vi "Model OPCUA Check Status.vi"(8 "error in (no error)":errorcluster, 11 "Model_AMC in":refnum<class "Model_AMC.lvclass">) -> (0 "error out":errorcluster, 3 "Model_AMC out":refnum<class "Model_AMC.lvclass">)   [LabVIEW 2021, in "Model_AMC.lvclass"]
uses:
  Model_AMC.lvclass
  Model_AMC.lvclass/Model_AMC.ctl
  <userlib>/John_Lib/AMC_FW/AMC_FW.lvlib
  <userlib>/John_Lib/OPCUA/OPCUA.lvclass
  1a8ff785-ae6d-495a-9cae-a72b057f70a7.vi
  d4dfea47-cd05-4011-96e4-e19734fac517.vi
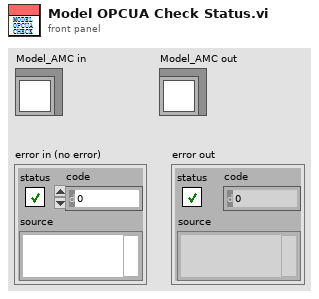
[diagram p1: front panel]
types:
  T1 = typedef "AMC_FW.lvlib/Queue.ctl" = cluster{"Q":T2, "Name":string}
  T2 = typedef "AMC_FW.lvlib/Message Queue.ctl" = refnum<queue>
  T3 = typedef "Model_AMC.lvclass/DVR.ctl" = cluster{"JKI_Network_Streams":refnum<class "NetworkConnection.lvclass">, "AMC Q":T4}
  T4 = typedef "Model_AMC.lvclass/AMC Q.ctl" = cluster{"Main":T1, "OPCUA":T1, "NetworkSteam":T1}
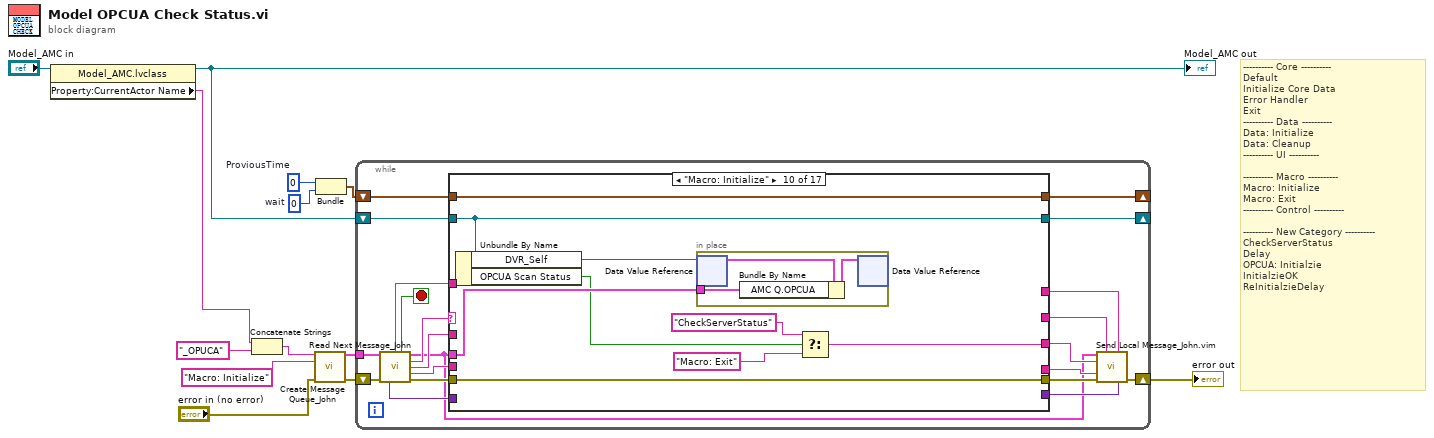
[diagram p0: block diagram]
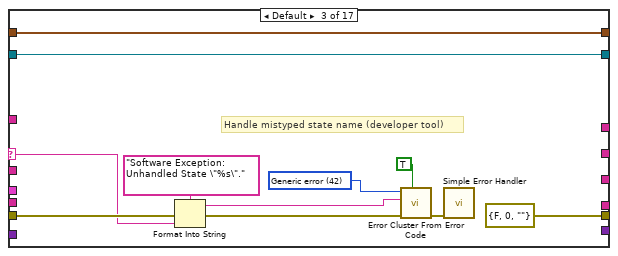
[diagram p4: hidden frame]
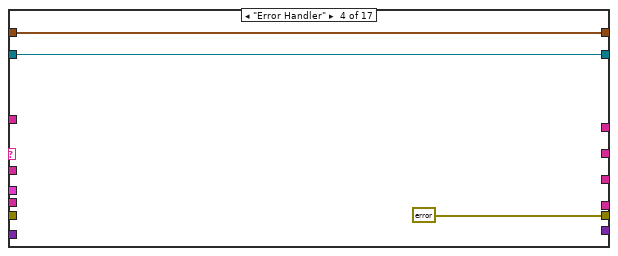
[diagram p5: hidden frame]
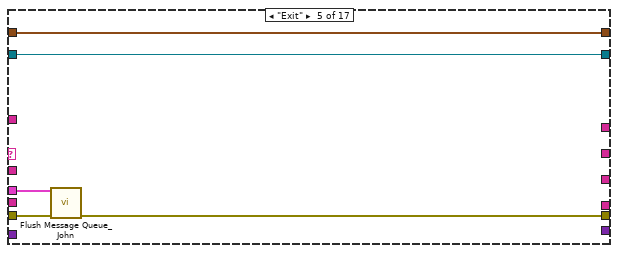
[diagram p6: hidden frame]
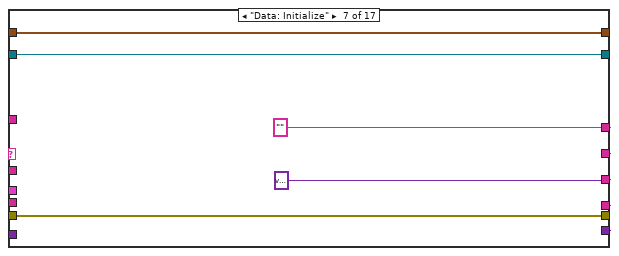
[diagram p8: hidden frame]
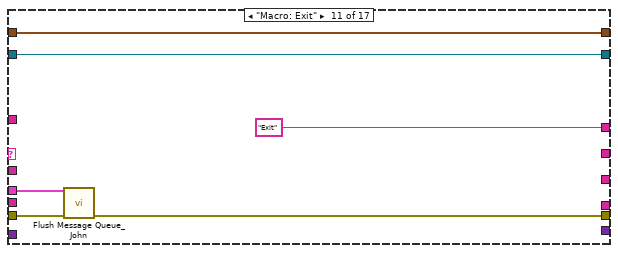
[diagram p11: hidden frame]
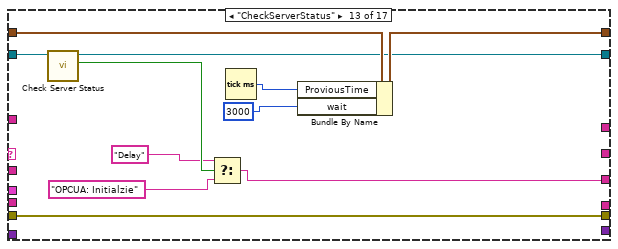
[diagram p13: hidden frame]
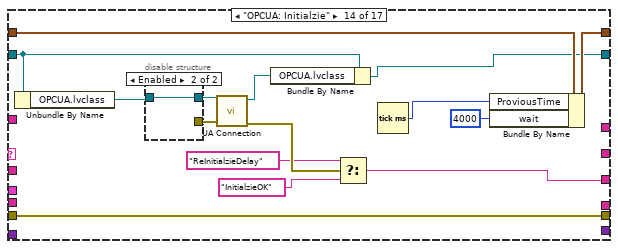
[diagram p14: hidden frame]
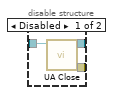
[diagram p15: hidden frame]
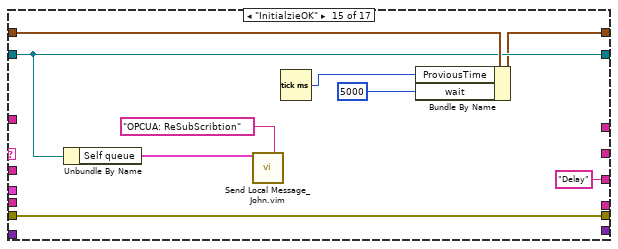
[diagram p16: hidden frame]
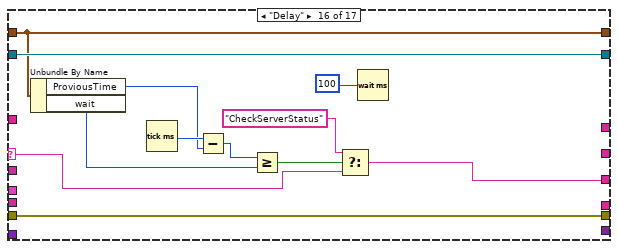
[diagram p17: hidden frame]
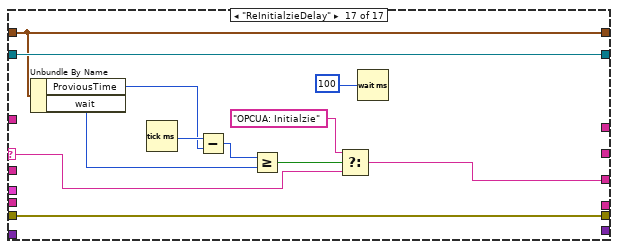
[diagram p18: hidden frame]
diagram:
  w13 = u32 0  # wait
  w6 = u32 0  # ProviousTime
  # "---------- Core ----------\nDefault\nInitialize Core Data\nError Handler\nExit\n---------- Data ----------\nData: Initialize\nData: Cleanup\n---------- UI ----------\n\n---------- Macro ----------\nMacro: Initialize\nMacro: Exit\n---------- Control ----------\n\n---------- New Category ----------\nCheckServerStatus\nDelay\nOPCUA: Initialzie\nInitialzieOK\nReInitialzieDelay"
  n1 = property class="Model_AMC.lvclass"(reference="Model_AMC in") -> (reference out=w2:refnum<class "Model_AMC.lvclass">, "Property:CurrentActor Name"=w1:string)  [unwired: 1 in, 1 out]
  "Model_AMC out" <- w2
  n2 = Concatenate Strings(w1, "_OPUCA" ("string")) -> (w8:string)
  n3 = call <userlib>:"Create Message Queue_John.vi"("message queue name"=w8, "initial message names"="Macro: Initialize", "error in"="error in (no error)") -> ("message queue out"=w10:T1, "error out"=w11:errorcluster)  [unwired: 11 in]
  n4 = Bundle("ProviousTime"=w6, "wait"=w13) -> (w7:cluster{"ProviousTime":u32, "wait":u32})  [unwired: 1 in]
  n5 = while {
    shift-right: [w25] -> w3
    shift-left: w11 -> [w33]
    shift-right: [w34] -> _
    shift-left: w2 -> [w27]
    tunnel: w10 -> [w30]
    shift-right: [w15] -> _
    shift-left: w7 -> [w16]
    stop <- w17 stop-if-true
    n6 = call <userlib>:"Read Next Message_John.vi"("Queue In"=w30, "error in"=w33) -> ("Previous State + Arguments"=w26:string, "exit process?"=w17:bool, "Queue Out"=w14:T1, "Current State"=w31:string, "Arguments"=w29:string, "message value"=w28:string, "variant"=w18:variant, "error out"=w32:errorcluster)  [unwired: 4 in, 2 out]
    n7 = case shown="\"Macro: Initialize\"" w31 {
      selector: w31 -> [_ _ w46 _ _ _ _ _ _ _ _ _ _ _ _ w137 w149]
      tunnel: w14 -> [_ _ _ _ w57 _ _ _ _ w78 w91 _ _ _ _ _ _]
      tunnel: w28 -> [_ _ _ _ _ _ _ _ _ _ _ _ _ _ _ _ _]
      tunnel: [w36 w40 errorcluster {"status"=FALSE, "code"=0, "source"=""} ("error out") errorcluster {"status"=FALSE, "code"=0, "source"=""} ("error out") w58 w61 w67 w69 w72 w82 w89 w94 w100 w120 w133 w145 w157] -> w24
      tunnel: w32 -> [w36 w40 w47 _ w59 w61 w67 w69 w72 w82 w90 w94 w100 w120 w133 w145 w157]
      tunnel: w27 -> [w37 w39 w43 w54 w56 w62 w65 w70 w73 w80 w88 w93 w105 w107 w131 w144 w156]
      tunnel: [w37 w39 w43 w54 w56 w62 w65 w70 w73 w80 w88 w93 w101 w106 w131 w144 w156] -> w34
      tunnel: w29 -> [_ _ _ _ _ _ _ _ _ _ _ _ _ _ _ _ _]
      tunnel: w26 -> [_ _ _ _ _ _ _ _ _ _ _ _ _ _ _ _ _]
      tunnel: [_ _ _ _ _ _ w66 _ _ _ _ _ _ _ _ _ _] -> w23
      tunnel: [_ _ _ _ _ _ w66 _ _ _ "Exit" _ _ _ _ _ _] -> w22
      tunnel: [_ _ _ _ _ _ w66 _ _ w75 _ _ w95 w113 "Delay" ("Previous State + Arguments") w136 w148] -> w21
      tunnel: [_ _ _ _ _ _ w66 _ _ _ _ _ _ _ _ _ _] -> w20
      tunnel: [_ _ _ _ _ _ variant ("variant") _ _ _ _ _ _ _ _ _ _] -> w19
      tunnel: w18 -> [_ _ _ _ _ _ _ _ _ _ _ _ _ _ _ _ _]
      tunnel: w16 -> [w35 w38 w41 w52 w55 w60 w63 w68 w71 w81 w86 w92 w104 w119 w132 w143 w155]
      tunnel: [w35 w38 w41 w52 w55 w60 w63 w68 w71 w81 w86 w92 w103 w112 w127 w143 w155] -> w15
      frame "", "Idle" {
      }
      frame "---------- Core ----------" {
      }
      frame Default {
        w49 = 42 items=["No error", "Argument error", "Memory is full", "Out of zone", "End of file", "File already open", "Generic file I/O error", "File not found", "File permission error", "Disk is full", "Duplicate path", "Too many files open", "System feature not enabled", "Resource file not found", "Cannot add resource", "Resource not found", "Image not found", "Image memory error", "Pen does not exist", "Config type invalid", "Config token not found", "Config parse error", "Config memory error", "Bad external code format", "Bad external code offset", "External code not present", "Null window", "Destroy window error", "Null menu", "Print aborted", "Bad print record", "Print driver error", "Windows error during printing", "Memory error during printing", "Print dialog error", "Generic print error", "Invalid device refnum", "Device not found", "Device parameter error", "Device unit error", "Cannot open device", "Device call aborted", "Generic error", "Cancelled by user", "Object ID too low", "Object ID too high", "Object not in heap", "Unknown heap", "Unknown object (invalid DefProc)", "Unknown object (DefProc not in table)", "Message out of range", "Invalid (null) method", "Unknown message", "Manager call not supported", "Bad address", "Network operation in progress", "Network operation timed out", "Connection is busy", "Network attribute not supported", "Network error", "Address in use", "System out of memory", "Connection aborted", "Connection refused", "Not connected", "Already connected", "Connection closed", "Initialization error (interapplication manager)", "Bad occurrence", "Wait on unbound occurrence handler", "Occurrence queue overflow", "Datalog type conflict", "Unused", "Unrecognized type (interapplication manager)", "Memory corrupt", "Failed to make temporary DLL", "Old CIN version", "Drag socket not found", "Failed to load drop-object", "Failed to register OLE object", "Failed to release OLE object", "Format specifier type mismatch", "Unknown format specifier", "Too few format specifiers", "Too many format specifiers", "Scan failed", "Newer CIN version", "Error converting to variant", "Runtime menu error", "Password tampered", "Variant attribute not found", "Incompatible variant data type", "Event data is not available", "Event Store is not present", "Occurrence is not found", "Event Queue is not created", "Event info is not available", "Refnum passed is NULL", "Error retrieving Class GUID", "Error retrieving CoClass GUID", "Error retrieving TypeLib GUID.", "Bad built application magic bytes.", "Specific driver is different from the specific driver associated with the Logical Name.", "There is no session opened to the class driver.", "Max Error", "MAX - Error with config objects", "MAX - Error loading configuration", "MAX - Group not supported"]
        # "Handle mistyped state name (developer tool)"
        n8 = Format Into String(format string="Software Exception: Unhandled State \"%s\"." ("message"), error in=w47, w46) -> (resulting string=w42:string, error out=w50:errorcluster)  [unwired: 1 in]
        n9 = call <vilib>:"Error Cluster From Error Code.vi"("show call chain? (False)"=TRUE, "error in (no error)"=w50, "error message (\"\")"=w42, "error code (0)"=w49) -> ("error out"=w45:errorcluster)  [unwired: 5 in]
        n10 = call <vilib>:"Simple Error Handler.vi"("error in (no error)"=w45) -> ()  [unwired: 4 in, 5 out]
      }
      frame "Error Handler" {
      }
      frame "Exit" {
        n11 = call <userlib>:"Flush Message Queue_John.vi"("Queue In"=w57, "error in"=w59) -> ("error out"=w58:errorcluster)  [unwired: 11 in, 2 out]
      }
      frame "---------- Data ----------" {
      }
      frame "Data: Initialize" {
        w66 = "" ("Elements in Front")
      }
      frame "---------- UI ----------" {
      }
      frame "---------- Macro ----------" {
      }
      frame "Macro: Initialize" {
        n12 = Unbundle By Name(w80) -> ("DVR_Self"=w79:refnum<data-value>, "OPCUA Scan Status"=w77:bool)
        n13 = in-place {
          in-place-border: w78 -> [w83]
          n14 = in-place-dvr #1(w79) -> (w85:T3)  [unwired: 1 out]
          n15 = Bundle By Name(cluster=w85, "AMC Q.OPCUA"=w83) -> (w84:T3)
          n16 = in-place-dvr #1(w84) -> ()  [unwired: 2 out]
        }
        n17 = Select(t="CheckServerStatus", s=w77, f="Macro: Exit") -> (s? t:f=w75:string)
      }
      frame "Macro: Exit" {
        n18 = call <userlib>:"Flush Message Queue_John.vi"("Queue In"=w91, "error in"=w90) -> ("error out"=w89:errorcluster)  [unwired: 11 in, 2 out]
      }
      frame "---------- Control ----------" {
      }
      frame "CheckServerStatus" {
        n19 = call "Check Server Status.vi"("Model_AMC in"=w105) -> ("T: OK"=w99:bool, "Model_AMC out"=w101:refnum<class "Model_AMC.lvclass">)  [unwired: 8 in, 1 out]
        n20 = Select(t="Delay" ("Elements in Front"), s=w99, f="OPCUA: Initialzie" ("Elements in Front")) -> (s? t:f=w95:string)
        n21 = Tick Count (ms)() -> (millisecond timer value=w102:u32)
        n22 = Bundle By Name(cluster=w104, "ProviousTime"=w102, "wait"=u32 3000 ("t")) -> (w103:cluster{"ProviousTime":u32, "wait":u32})
      }
      frame "OPCUA: Initialzie" {
        n23 = Unbundle By Name(w107) -> ("OPCUA.lvclass"=w109:refnum<class "OPCUA.lvclass">)
        n24 = disable-structure shown="Enabled" {
          disable-tunnel: [w123 _] -> w118
          disable-tunnel: w109 -> [w122 w124]
          disable-tunnel: [w121 w124] -> w117
          frame Disabled {
            n25 = call <userlib>:"UA Close.vi"("OPCUA in"=w122) -> ("error out"=w123:errorcluster, "OPCUA out"=w121:refnum<class "OPCUA.lvclass">)  [unwired: 9 in]
          }
          frame Enabled {
          }
        }
        n26 = call <userlib>:"UA Connection.vi"("error in (no error)"=w118, "OPCUA in"=w117) -> ("error out"=w116:errorcluster, "OPCUA out"=w108:refnum<class "OPCUA.lvclass">)  [unwired: 8 in]
        n27 = Bundle By Name(cluster=w107, "OPCUA.lvclass"=w108) -> (w106:refnum<class "Model_AMC.lvclass">)
        n28 = Select(t="ReInitialzieDelay" ("string"), s=w116, f="InitialzieOK") -> (s? t:f=w113:string)
        n29 = Tick Count (ms)() -> (millisecond timer value=w111:u32)
        n30 = Bundle By Name(cluster=w119, "ProviousTime"=w111, "wait"=u32 4000) -> (w112:cluster{"ProviousTime":u32, "wait":u32})
      }
      frame "InitialzieOK" {
        n31 = Unbundle By Name(w131) -> ("Self queue"=w130:T1)
        n32 = call "Send Local Message_John.vim"("Queue In"=w130, "Elements in Front"="OPCUA: ReSubScribtion") -> ()  [unwired: 11 in, 3 out]
        n33 = Tick Count (ms)() -> (millisecond timer value=w125:u32)
        n34 = Bundle By Name(cluster=w132, "ProviousTime"=w125, "wait"=u32 5000) -> (w127:cluster{"ProviousTime":u32, "wait":u32})
      }
      frame "Delay" {
        n35 = Unbundle By Name(w143) -> ("ProviousTime"=w141:u32, "wait"=w134:u32)
        n36 = Tick Count (ms)() -> (millisecond timer value=w142:u32)
        n37 = Subtract(x=w142, y=w141) -> (x-y=w140:u32)
        n38 = Greater Or Equal?(x=w140, y=w134) -> (x >= y?=w139:bool)
        n39 = Select(t="CheckServerStatus" ("Previous State + Arguments"), s=w139, f=w137) -> (s? t:f=w136:string)
        n40 = Wait (ms)(milliseconds to wait=u32 100) -> ()  [unwired: 1 out]
      }
      frame "ReInitialzieDelay" {
        n41 = Unbundle By Name(w155) -> ("ProviousTime"=w153:u32, "wait"=w146:u32)
        n42 = Tick Count (ms)() -> (millisecond timer value=w154:u32)
        n43 = Subtract(x=w154, y=w153) -> (x-y=w152:u32)
        n44 = Greater Or Equal?(x=w152, y=w146) -> (x >= y?=w151:bool)
        n45 = Select(t="OPCUA: Initialzie" ("Previous State + Arguments"), s=w151, f=w149) -> (s? t:f=w148:string)
        n46 = Wait (ms)(milliseconds to wait=u32 100) -> ()  [unwired: 1 out]
      }
    }
    n47 = call "Send Local Message_John.vim"("Queue In"=w14, "receiver process (\"\" - local)"=w23, "Elements in Front"=w22, "Elements at Back"=w21, "message value"=w20, "error in"=w24, "variant"=w19) -> ("error out"=w25:errorcluster)  [unwired: 6 in, 2 out]
  }
  "error out" <- w3
